vi "Error Magic.vi"(6 "Variant in":variant, 7 "Shift Pressed?":bool, 8 "error in (no error)":errorcluster, 10 "QD Combo Box Ref":refnum<vi>, 11 "QD Launch VI Ref":refnum<vi>) -> (0 "error out":errorcluster, 4 "Variant out":variant)   [LabVIEW 2017]
doc: "Ensures that there are Error In and Error Out controls on the front panel, positioned above the origin and that they are attached to the connector pane terminals.\n\nDefault Shortcut - [E]"
panel:
  in  "Undo Name":string="Quick Drop Keyboard Shortcut"
  # "Do not change the connector pane of this VI.\n\nSee the block diagram for directions on how to use this template."
  # "Specify the name of the Undo transaction"
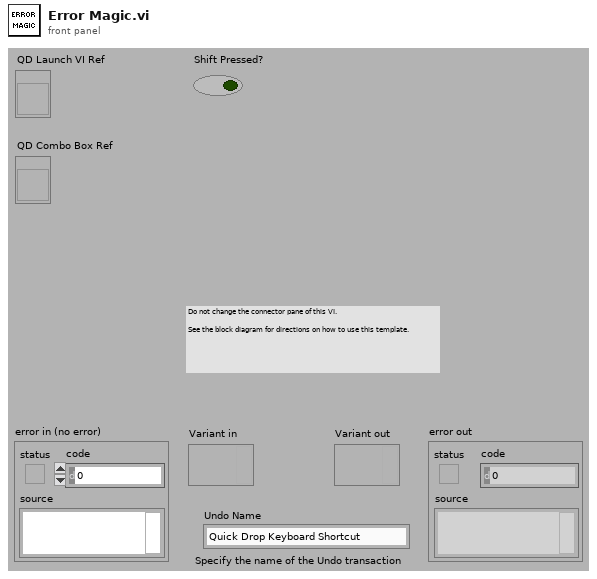
[diagram p1: front panel]
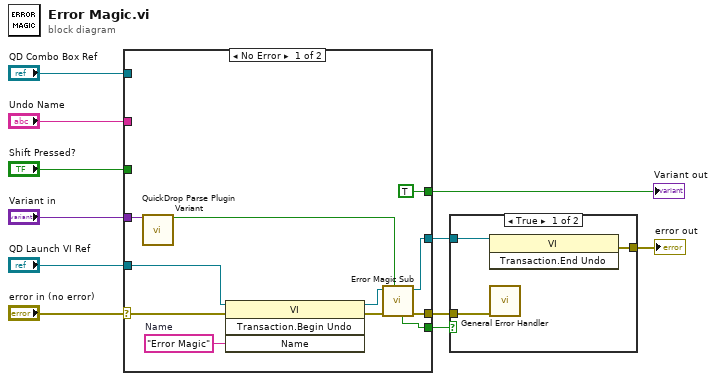
[diagram p0: block diagram]
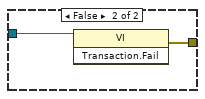
[diagram p2: hidden frame]
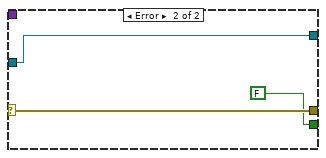
[diagram p3: hidden frame]
diagram:
  n1 = case shown="No Error" "error in (no error)" {
    selector: "error in (no error)" -> [w21 w25]
    tunnel: [w17 w25] -> w4
    tunnel: "QD Launch VI Ref" -> [w20 w24]
    tunnel: "Shift Pressed?" -> [_ _]
    tunnel: "QD Combo Box Ref" -> [_ _]
    tunnel: "Variant in" -> [w22 _]
    tunnel: "Undo Name" -> [_ _]
    tunnel: [TRUE _] -> w5
    tunnel: [w12 FALSE] -> w2
    tunnel: [w14 w24] -> w1
    frame No Error {
      w15 = "Error Magic"  # Name
      n2 = call <vilib>:"QuickDrop Parse Plugin Variant.vi"("QDKS Variant in"=w22) -> ("QD Launch VI Panel?"=w13:bool)  [unwired: 12 in, 2 out]
      n3 = invoke class="VI" method="Transaction.Begin Undo"(reference=w20, error in=w21, "Name"=w15) -> (reference out=w16:refnum<vi>, error out=w18:errorcluster)  [unwired: 1 in, 2 out]
      n4 = call "Error Magic Sub.vi"("QD Launch VI Panel?"=w13, "error in (no error)"=w18, "VI in"=w16) -> ("error out"=w17:errorcluster, "VI out"=w14:refnum<vi>, "Completed"=w12:bool)  [unwired: 6 in]
    }
    frame Error {
    }
  }
  "Variant out" <- w5
  n5 = case shown="True" w2 {
    tunnel: w1 -> [w27 w29]
    tunnel: [w28 w30] -> w3
    tunnel: w4 -> [w26 _]
    frame True {
      n6 = invoke class="VI" method="Transaction.End Undo"(reference=w27) -> (error out=w28:errorcluster)  [unwired: 2 in, 2 out]
      n7 = call <vilib>:"General Error Handler.vi"("error in (no error)"=w26) -> ()  [unwired: 10 in, 5 out]
    }
    frame False {
      n8 = invoke class="VI" method="Transaction.Fail"(reference=w29) -> (error out=w30:errorcluster)  [unwired: 2 in, 2 out]
    }
  }
  "error out" <- w3
